vi "Get Register Address Field Width.vi"(8 "error in (no error)":errorcluster, 11 "RFFE Extended Command in":refnum<class "RFFE Extended Command.lvclass">) -> (0 "error out":errorcluster, 2 "Register Address Field Width":i32, 3 "RFFE Extended Command out":refnum<class "RFFE Extended Command.lvclass">)   [LabVIEW 2018, in "MIPI RFFE API.lvlib" / "RFFE Extended Command.lvclass"]
uses:
  RFFE Extended Command.lvclass
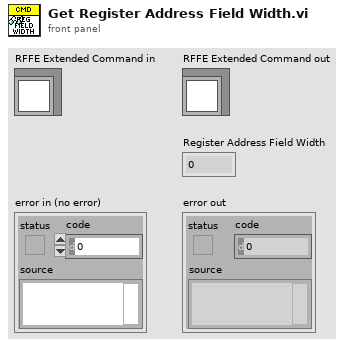
[diagram p1: front panel]
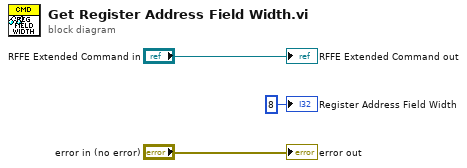
[diagram p0: block diagram]
diagram:
  "error out" <- "error in (no error)"
  "RFFE Extended Command out" <- "RFFE Extended Command in"
  "Register Address Field Width" <- 8 ("Register Address Field Width")
